vi "SetSpecParameters.vi"(0 "Spectroscopy Cluster":T1={"Mode"=0, "Start [a.u.]"=-inf, "End [a.u.]"=-inf, "Points"=-2147483648, "Repeat"=-2147483648, "Fwd/Bwd"=FALSE, "Delay"=-inf, "Preferences Button"=FALSE, "DAC"=0, "Avg Time"=-inf} {"Avg Time" format="%#_g µs"; "DAC" items=["DAC 1"=0, "DAC 2"=1, "DAC 3"=2, "DAC 4"=3, "Z"=26, "Low Frequency"=27]; "Delay" format="%#_g µs"; "Mode" items=["Spectroscopy 1", "Spectroscopy 2", "Spectroscopy 3", "Calibration"]}, 5 "error in":T4) -> (14 "Output Cluster":T1={"Mode"=0, "Start [a.u.]"=-inf, "End [a.u.]"=-inf, "Points"=-2147483648, "Repeat"=-2147483648, "Fwd/Bwd"=FALSE, "Delay"=-inf, "Preferences Button"=FALSE, "DAC"=0, "Avg Time"=-inf} {"Avg Time" format="%#_g µs"; "DAC" items=["DAC 1"=0, "DAC 2"=1, "DAC 3"=2, "DAC 4"=3, "Z"=26, "Low Frequency"=27]; "Delay" format="%#_g µs"; "Mode" items=["Spectroscopy 1", "Spectroscopy 2", "Spectroscopy 3", "Calibration"]}, 19 "error out":T4)   [LabVIEW 2016]
doc: "This VI sets all parameters associated with spectroscopy mode. The input cluster contains the following:\n- DAC (integer) [DAC 1-DAC 4; Z; Low Frequency]\n- Mode (integer) [0-2 -- Spectroscopy1-3; 3 -- Calibration]\n- Start (float) [depends on DAC input: mV, Hz or degree]\n- End (float) [depends on DAC input: mV, Hz or degree]\n- Points (integer) [0 to 65535]\n- fwd (integer) [0 to 1]\n- Repeat (integer) [0 to 65535]\n- Delay in µs (float) [0 to 10000000]\n- Average Time in µs (float) [0 to 10000000]\nBy passing -Inf (float) or -2147483648 (integer) as input values, the corresponding parameter(s) will be read out."
uses:
  Controls/Spectroscopy_Parameters.ctl
  Controls/Spectroscopy-Mode_Selection.ctl
  Controls/Spec_DAC_Selection.ctl
  Controls/Error_Out.ctl
  Files_ASC500/DLL/ASC500_RemoteControlV27.dll
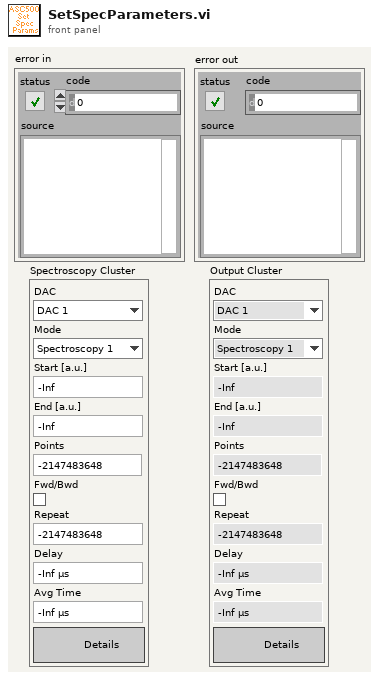
[diagram p1: front panel]
types:
  T1 = typedef "Spectroscopy_Parameters.ctl" = cluster{"Mode":T2, "Start [a.u.]":sgl, "End [a.u.]":sgl, "Points":i32, "Repeat":i32, "Fwd/Bwd":bool, "Delay":sgl, "Preferences Button":bool, "DAC":T3, "Avg Time":sgl}
  T2 = typedef "Spectroscopy-Mode_Selection.ctl" = u16
  T3 = typedef "Spec_DAC_Selection.ctl" = u16
  T4 = typedef "Error_Out.ctl" = errorcluster
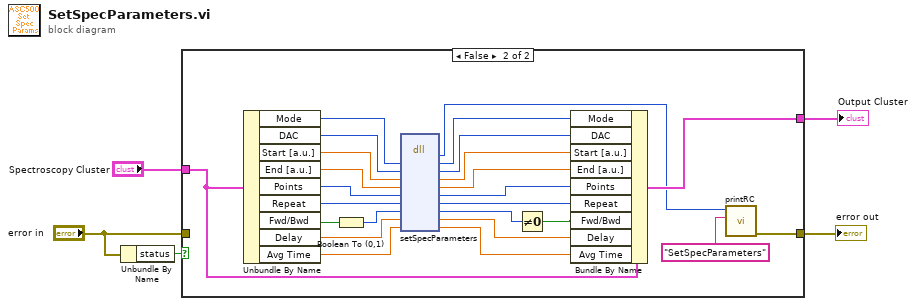
[diagram p0: block diagram]
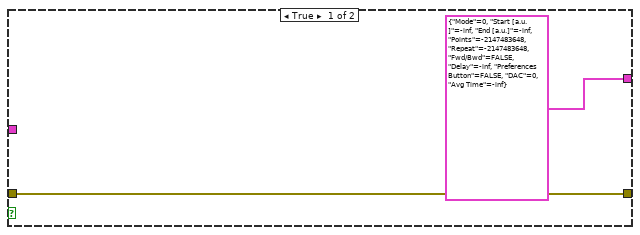
[diagram p2: hidden frame]
diagram:
  n1 = Unbundle By Name("error in") -> ("status"=w5:bool)
  n2 = case shown="False" w5 {
    tunnel: [w6 w24] -> w4
    tunnel: "Spectroscopy Cluster" -> [_ w29]
    tunnel: [T1 {"Mode"=0, "Start [a.u.]"=-inf, "End [a.u.]"=-inf, "Points"=-2147483648, "Repeat"=-2147483648, "Fwd/Bwd"=FALSE, "Delay"=-inf, "Preferences Button"=FALSE, "DAC"=0, "Avg Time"=-inf} ("Spectroscopy Cluster") w25] -> w2
    tunnel: "error in" -> [w6 _]
    frame True {
    }
    frame False {
      n3 = Unbundle By Name(w29) -> ("Mode"=w12:T2, "DAC"=w13:T3, "Start [a.u.]"=w32:sgl, "End [a.u.]"=w31:sgl, "Points"=w30:i32, "Repeat"=w19:i32, "Fwd/Bwd"=w14:bool, "Delay"=w20:sgl, "Avg Time"=w9:sgl)
      n4 = Boolean To (0,1)(Boolean=w14) -> (0, 1=w18:i16)
      n5 = dll-call lib="G:/SCMOperations/Share/ELE/Produkt Information/ASC500/04 Remote Control/02 development versions/2018Nov06/Files_ASC500/DLL/ASC500_RemoteControlV27.dll" fn="setSpecParameters"("Mode"=w12, "DAC"=w13, "Start"=w32, "End"=w31, "Points"=w30, "Repeat"=w19, "fbwd"=w18, "Delay"=w20, "avgTime"=w9) -> ("return type"=w23:i32, "Mode"=w11:i32, "DAC"=w10:i32, "Start"=w28:sgl, "End"=w27:sgl, "Points"=w26:i32, "Repeat"=w15:i32, "fbwd"=w16:i32, "Delay"=w21:sgl, "avgTime"=w8:sgl)  [unwired: 3 in, 2 out]
      n6 = Not Equal To 0?(x=w16) -> (x != 0?=w17:bool)
      n7 = Bundle By Name(cluster=w29, "Mode"=w11, "DAC"=w10, "Start [a.u.]"=w28, "End [a.u.]"=w27, "Points"=w26, "Repeat"=w15, "Fwd/Bwd"=w17, "Delay"=w21, "Avg Time"=w8) -> (w25:T1)
      n8 = call "printRC.vi"("additional information"="SetSpecParameters", "RC"=w23) -> ("error out"=w24:T4)  [unwired: 9 in]
    }
  }
  "error out" <- w4
  "Output Cluster" <- w2
